vi "Init.vi"(8 "error in (no error)":errorcluster, 10 "index":i32, 11 "IC_2D":refnum<class "NI_IC_2D.lvclass">) -> (0 "error out":errorcluster, 3 "initialized IC_2D":refnum<class "NI_IC_2D.lvclass">)   [LabVIEW 2017, in "NI_PDE.lvlib" / "NI_IC_2D.lvclass"]
uses:
  <vilib>/gmath/pde.llb/ICClass/IC_2D/NI_IC_2D.lvclass
  <vilib>/gmath/pde.llb/ICClass/Class Type.ctl
  <vilib>/gmath/pde.llb/ICClass/NI_IC.lvclass
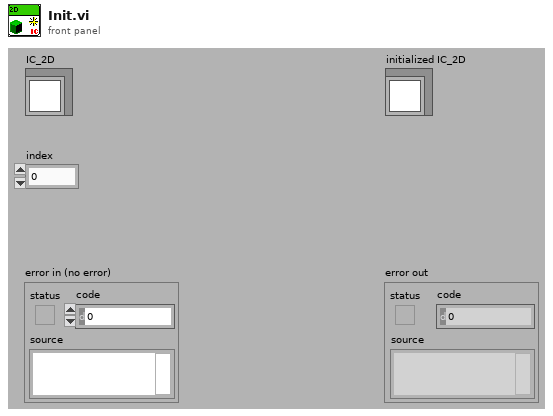
[diagram p1: front panel]
types:
  T1 = typedef "NI_PDE.lvlib/NI_IC.lvclass/Class Type.ctl" = i32
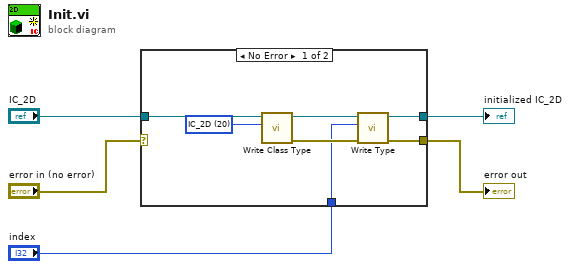
[diagram p0: block diagram]
diagram:
  n1 = case shown="No Error" "error in (no error)" {
    selector: "error in (no error)" -> [_ w14]
    tunnel: "IC_2D" -> [w12 w13]
    tunnel: [w8 w13] -> w2
    tunnel: [w7 w14] -> w4
    tunnel: "index" -> [w6 _]
    frame No Error {
      w11 = T1 20 items=["IC"=0, "IC_1D"=10, "IC_1D_Numeric"=11, "IC_1D_VIRef"=12, "IC_2D"=20, "IC_2D_Numeric"=21, "IC_2D_VIRef"=22] ("IC class type")
      n2 = call-dynamic "Write Class Type.vi"("IC class type"=w11, "IC.lvclass in"=w12) -> ("error out"=w9:errorcluster, "IC.lvclass out"=w10:refnum<class "NI_IC_2D.lvclass">)  [unwired: 1 in, 7 out]
      n3 = call-dynamic "Write Type.vi"("error in (no error)"=w9, "IC type"=w6, "IC.lvclass in"=w10) -> ("error out"=w7:errorcluster, "IC.lvclass out"=w8:refnum<class "NI_IC_2D.lvclass">)  [unwired: 7 out]
    }
    frame Error {
    }
  }
  "initialized IC_2D" <- w2
  "error out" <- w4
